vi "SA - Verify Sampling Rate Validity.vi"(0 "Time in":waveform(dbl)[](array[waveform]), 5 "error in (no error)":errorcluster, 6 "Nb Signals":i32) -> (14 "Time out":waveform(dbl)[](array[waveform]), 19 "error out":errorcluster)   [LabVIEW 2020, in "GSwFormDSP.lvclass"]
uses:
  GSwFormDSP.lvclass
  functions/Sampling Rate Fs.ctl
  functions/Attribute List.ctl
panel:
  out "Signals Name":string
  in  "Cancel":bool
  in  "User Input Fs":T1 caption="Sampling Rate"
  # "The following signal does NOT have an assign sampling rate."
  # "Please assign a sampling rate."
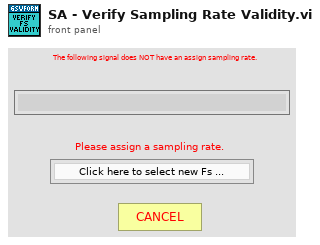
[diagram p1: front panel]
types:
  T1 = typedef "GSwFormDSP.lvclass/Sampling Rate Fs.ctl" = enum16{"Click here to select new Fs ...", "1 Hz", "2 Hz", "4 Hz", "8 Hz", "16 Hz", "32 Hz", "64 Hz", "128 Hz", "256 Hz", "512 Hz", "1024 Hz", "2048 Hz", "4096 Hz", "8 kHz", "8192 Hz", "11025 Hz", "16 kHz", "16384 Hz", "22050 Hz", "32768 Hz", "44100 Hz", "48000 Hz"}
  T2 = typedef "GSwFormDSP.lvclass/Attribute List.ctl" = string
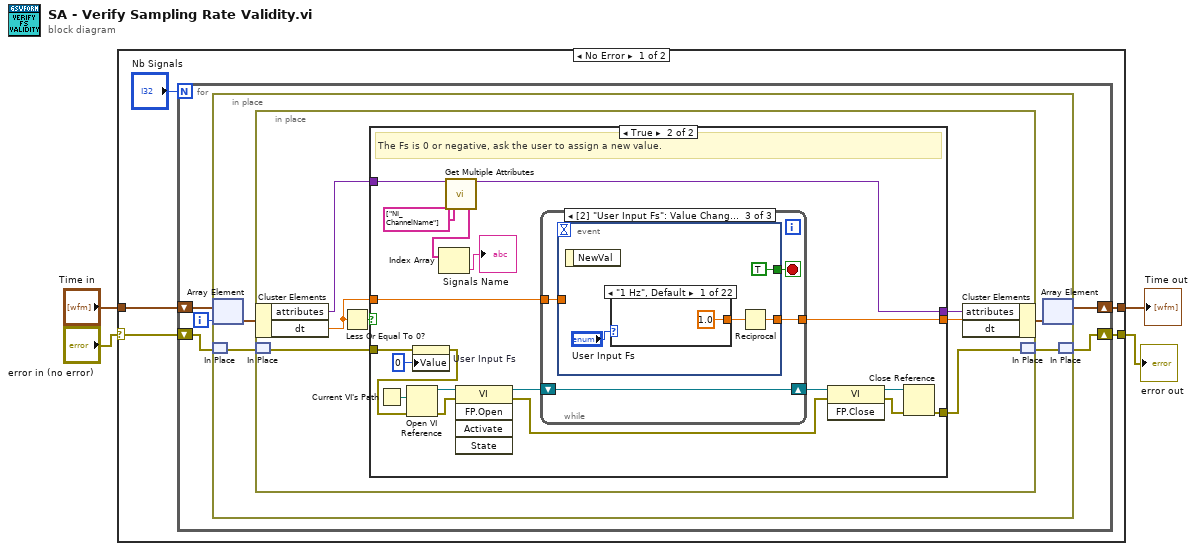
[diagram p0: block diagram]
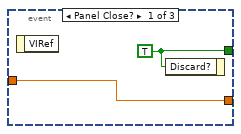
[diagram p3: hidden frame]
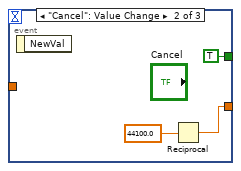
[diagram p4: hidden frame]
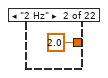
[diagram p5: hidden frame]
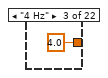
[diagram p6: hidden frame]
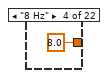
[diagram p7: hidden frame]
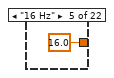
[diagram p8: hidden frame]
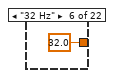
[diagram p9: hidden frame]
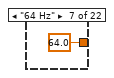
[diagram p10: hidden frame]
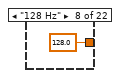
[diagram p11: hidden frame]
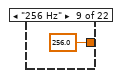
[diagram p12: hidden frame]
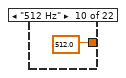
[diagram p13: hidden frame]
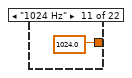
[diagram p14: hidden frame]
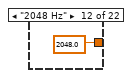
[diagram p15: hidden frame]
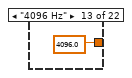
[diagram p16: hidden frame]
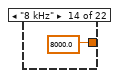
[diagram p17: hidden frame]
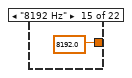
[diagram p18: hidden frame]
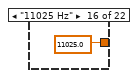
[diagram p19: hidden frame]
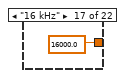
[diagram p20: hidden frame]
diagram:
  n1 = case shown="No Error" "error in (no error)" {
    selector: "error in (no error)" -> [w6 w84]
    tunnel: [w7 w84] -> w3
    tunnel: [w8 w83] -> w1
    tunnel: "Time in" -> [w9 w83]
    frame No Error {
      n2 = for {
        N: "Nb Signals" -> [_]
        shift-right: [w10] -> w8
        shift-left: w9 -> [w14]
        shift-right: [w11] -> w7
        shift-left: w6 -> [w12]
        i -> [w13]
        n3 = in-place {
          n4 = in-place-array #1(w14, w13) -> (w18:waveform(dbl))
          n5 = in-place-match #2(w12) -> (w17:errorcluster)
          n6 = in-place {
            n7 = in-place-cluster #3(w18) -> ("attributes"=w22:variant, "dt"=w23:dbl)
            n8 = in-place-match #4(w17) -> (w19:errorcluster)
            n9 = Less Or Equal To 0?(x=w23) -> (x <= 0?=w25:bool)
            n10 = case shown="True" w25 {
              tunnel: [w28 w47] -> w24
              tunnel: w23 -> [w28 w46]
              tunnel: w22 -> [w27 w45]
              tunnel: [w27 w43] -> w21
              tunnel: [w26 w32] -> w20
              tunnel: w19 -> [w26 w30]
              frame False {
                # "The sampling rate seems OK, so do nothing."
              }
              frame True {
                # "The Fs is 0 or negative, ask the user to assign a new value."
                n11 = Current VI's Path() -> (path=w40:path)
                n12 = property on="User Input Fs" class="Enum (strict)"(error in=w30, "Value"=0) -> (error out=w29:errorcluster)  [unwired: 1 in, 1 out]
                n13 = Open VI Reference(vi path=w40, error in (no error)=w29) -> (vi reference=w39:refnum<vi>, error out=w38:errorcluster)  [unwired: 4 in]
                n14 = call "Get Multiple Attributes.vi"("Attributes IN"=w45, "Attribute List"=T2[] ["NI_ChannelName"]) -> ("Values"=w42:string[], "Attributes OUT"=w43:variant)  [unwired: 16 in]
                n15 = Index Array(array=w42) -> (element=→"Signals Name":string)  [unwired: 1 in]
                n16 = invoke class="VI" method="FP.Open"(reference=w39, error in=w38) -> (reference out=w35:refnum<vi>, error out=w33:errorcluster)  [unwired: 3 in, 3 out]
                n17 = while {
                  tunnel: [w50] -> w47
                  tunnel: w46 -> [w49]
                  shift-right: [w48] -> w34
                  shift-left: w35 -> [w48]
                  stop <- w51 stop-if-true
                  n18 = event shown="[2] \"User Input Fs\": Value Change" {
                    selector: _ -> [_ _ _]
                    dyn-events: _ -> [_ _ _]
                    timeout: _ -> [_ _ _]
                    tunnel: [w53 TRUE ("Discard?") TRUE ("Discard?")] -> w51
                    tunnel: [w52 w54 w57] -> w50
                    tunnel: w49 -> [w52 _ _]
                    event Panel Close? {
                      w53 = TRUE ("Discard?")
                      n19 = event-data() -> ()  [unwired: 1 in, 1 out]
                      n20 = event-data("Discard?"=w53) -> ()  [unwired: 1 in, 1 out]
                    }
                    event "Cancel": Value Change {
                      n21 = event-data() -> ()  [unwired: 1 in, 1 out]
                      n22 = Reciprocal(x=44100.0) -> (1/x=w54:dbl)
                    }
                    event Value Change {
                      n23 = event-data() -> ()  [unwired: 1 in, 1 out]
                      n24 = case shown="\"1 Hz\", Default" "User Input Fs" {
                        tunnel: [1.0 2.0 4.0 8.0 16.0 32.0 64.0 128.0 256.0 512.0 1024.0 2048.0 4096.0 8000.0 8192.0 11025.0 16000.0 16384.0 22050.0 32768.0 44100.0 48000.0] -> w58
                        frame "1 Hz", Default {
                        }
                        frame "2 Hz" {
                        }
                        frame "4 Hz" {
                        }
                        frame "8 Hz" {
                        }
                        frame "16 Hz" {
                        }
                        frame "32 Hz" {
                        }
                        frame "64 Hz" {
                        }
                        frame "128 Hz" {
                        }
                        frame "256 Hz" {
                        }
                        frame "512 Hz" {
                        }
                        frame "1024 Hz" {
                        }
                        frame "2048 Hz" {
                        }
                        frame "4096 Hz" {
                        }
                        frame "8 kHz" {
                        }
                        frame "8192 Hz" {
                        }
                        frame "11025 Hz" {
                        }
                        frame "16 kHz" {
                        }
                        frame "16384 Hz" {
                        }
                        frame "22050 Hz" {
                        }
                        frame "32768 Hz" {
                        }
                        frame "44100 Hz" {
                        }
                        frame "48000 Hz" {
                        }
                      }
                      n25 = Reciprocal(x=w58) -> (1/x=w57:dbl)
                    }
                  }
                }
                n26 = invoke class="VI" method="FP.Close"(reference=w34, error in=w33) -> (reference out=w36:refnum<vi>, error out=w37:errorcluster)  [unwired: 1 in, 1 out]
                n27 = Close Reference(reference=w36, error in (no error)=w37) -> (error out=w32:errorcluster)
              }
            }
            n28 = in-place-cluster #3("attributes"=w21, "dt"=w24) -> (w16:waveform(dbl))
            n29 = in-place-match #4(w20) -> (w15:errorcluster)
          }
          n30 = in-place-array #1(w16) -> (w10:waveform(dbl)[])  [unwired: 1 out]
          n31 = in-place-match #2(w15) -> (w11:errorcluster)
        }
      }
    }
    frame Error {
    }
  }
  "error out" <- w3
  "Time out" <- w1
